vi "RT_W&R_ADC_W_DAC.vi"() -> ()   [LabVIEW 2018]
uses:
  <vilib>/Platform/TimedLoop/XDataNode/timing_clust.ctl
  <vilib>/Platform/TimedLoop/XDataNode/nitl_modes.ctl
  <vilib>/Platform/TimedLoop/XDataNode/wakeup.ctl
  <vilib>/FPGAPlugInAG/myRIO-1900/niLvFpga_Open_myRIO-1900.vi
  <vilib>/rvi/interface/common/dynamic/niFpgaDynamicAddResources.vi
  <vilib>/Utility/error.llb/Error Cluster From Error Code.vi
  <vilib>/rvi/errors/niLvFpgaAdjustHostInterfaceError.vi
  <vilib>/FPGAPlugInAG/Dynamic/niLvFpga_Close_Dynamic.vi
  <vilib>/Platform/TimedLoop/XDataNode/XDataNode.xnode
  <vilib>/rvi/interface/nirviOpenFPGA/nirviOpenFPGA.xnode
  ASPE_SC_Amp_HS/FPGA Bitfiles/ASPESCAmpControl_FPGATarget_FPGASPIW&RADCWDA_vR5pGZ7Mmx4.lvbitx
  FPGA_SPI_W&R_ADC_W_DACs.vi
  <vilib>/rvi/interface/nirviReadWriteControl/nirviReadWriteControl.xnode
  <vilib>/rvi/interface/nirviCloseFPGA/nirviCloseFPGA.xnode
  <vilib>/Platform/TimedLoop/XDataNode/XDNodeRunTimeDep.lvlib
  NiFpgaLv.dll
  <vilib>/rvi/interface/Simulation/niFpgaSimulationCallBeginRW.vi
panel:
  out "Loop rate (kHz)":dbl
  in  "Stop Button":bool
  in  "CH1":bool[](array[boolean])=[FALSE, FALSE, FALSE, FALSE, FALSE, TRUE, FALSE, FALSE, FALSE, FALSE, FALSE, FALSE, FALSE, FALSE, FALSE, FALSE]
  in  "CH4":bool[](array[boolean])=[FALSE, FALSE, TRUE, TRUE, FALSE, TRUE, FALSE, FALSE, FALSE, FALSE, FALSE, FALSE, FALSE, FALSE, FALSE, FALSE]
  in  "CH3":bool[](array[boolean])=[FALSE, FALSE, TRUE, FALSE, FALSE, TRUE, FALSE, FALSE, FALSE, FALSE, FALSE, FALSE, FALSE, FALSE, FALSE, FALSE]
  in  "CH2":bool[](array[boolean])=[FALSE, FALSE, FALSE, TRUE, FALSE, TRUE, FALSE, FALSE, FALSE, FALSE, FALSE, FALSE, FALSE, FALSE, FALSE, FALSE]
  out "ADC 4":dbl(graph)=-2.0281672948105642
  out "ADC 3":dbl(graph)=-0.5364908372369804
  out "ADC 2":dbl(graph)=-0.0015258556235409
  out "ADC 1":dbl(graph)=-0.0015258556235409
  in  "us":u32=150
  out "Finished Late? [i-1]":bool
  # "You can read the voltage ouput of sensors in the following plots"
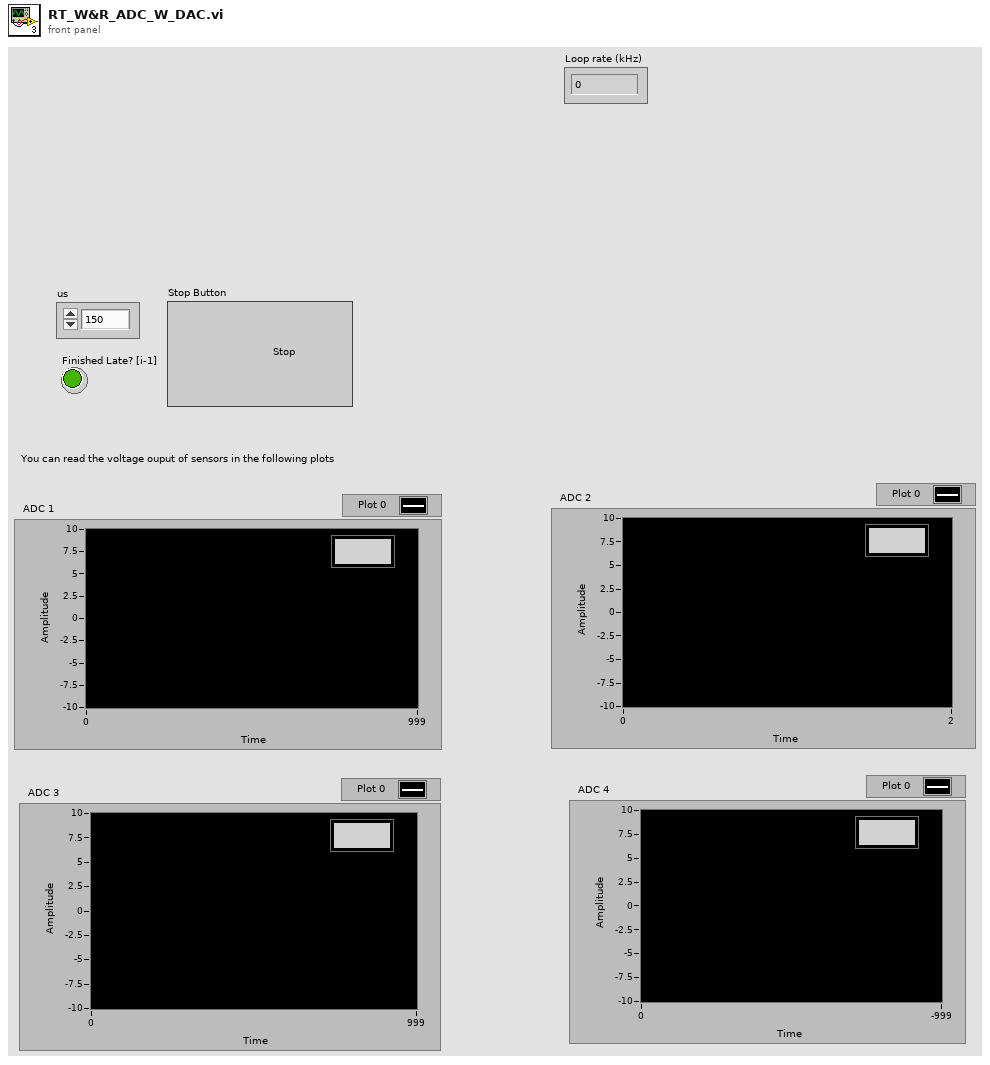
[diagram p1: front panel]
types:
  T1 = typedef "XDNodeRunTimeDep.lvlib/timing_clust.ctl" = cluster{"Expected End [f-1]":u64, "Actual End [f-1]":u64, "Finished Late? [f-1]":bool, "Expected End [i-1]":u64, "Actual End [i-1]":u64, "Finished Late? [i-1]":bool, "Expected Start [i]":u64, "Actual Start [i]":u64, "Expected Start [f]":u64, "Actual Start [f]":u64, "Source Name":string, "Structure Name":string, "Period":i64, "Deadline":i64, "Offset":i64, "Start":i64, "Priority":i32, "Timeout":i32, "Mode":T2, "Wakeup Reason":T3, "Error":errorcluster, "Source Type":string, "Secondary Source Type":string, "Global End Time":u64, "Global Start Time":u64, "Frame Duration":u64, "Iteration Duration":u64, "Assigned CPU":i32, "I/O Scan Engine Mode":u32}
  T2 = typedef "XDNodeRunTimeDep.lvlib/nitl_modes.ctl" = enum32{"No Change", "Process missed periods, maintain original phase", "Discard missed periods, maintain original phase", "Process missed periods, ignore original phase", "Discard missed periods, ignore original phase"}
  T3 = typedef "XDNodeRunTimeDep.lvlib/wakeup.ctl" = enum32{"Normal", "Aborted", "Asynchronous wakeup", "Timing source error", "Timed loop error", "Timeout"}
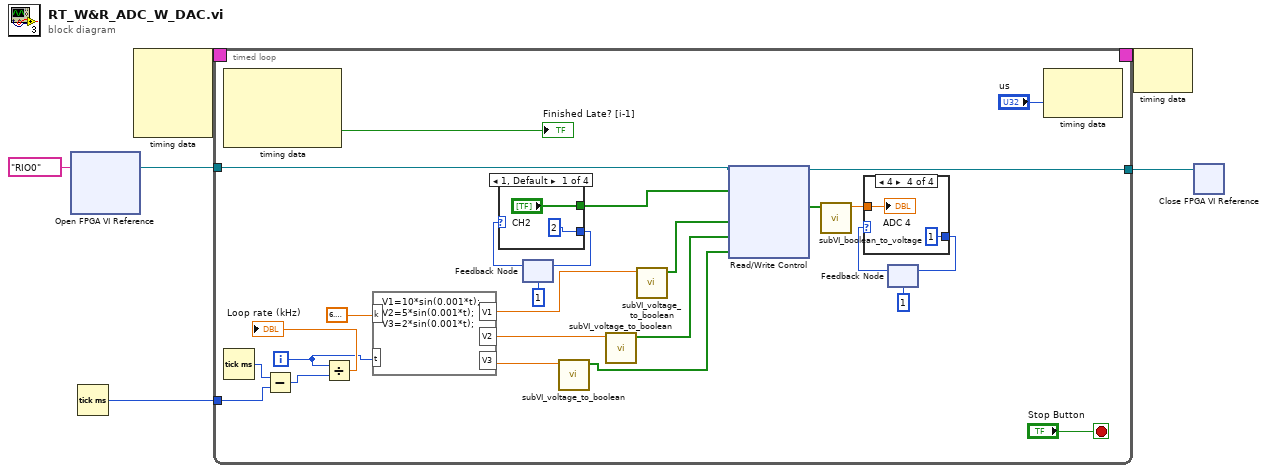
[diagram p0: block diagram]
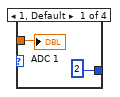
[diagram p2: hidden frame]
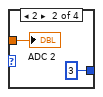
[diagram p3: hidden frame]
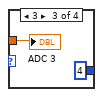
[diagram p4: hidden frame]
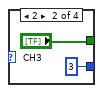
[diagram p5: hidden frame]
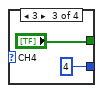
[diagram p6: hidden frame]
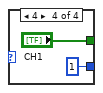
[diagram p7: hidden frame]
diagram:
  n1 = xnode "Open FPGA VI Reference"("resource name"=tag "RIO0") -> ("FPGA VI Reference Out"=w3:refnum<k20>)  [unwired: 1 in, 1 out]
  n2 = Tick Count (ms)() -> (millisecond timer value=w1:u32)
  n3 = node-c288() -> (w6:T1)  [unwired: 4 in]
  n4 = timed-loop {
    tunnel: w3 -> [w32]
    timing: w6 -> [_]
    timing-out: [_] -> w5
    tunnel: [w19] -> w4
    tunnel: w1 -> [w17]
    i -> [w13]
    stop <- "Stop Button" stop-if-true
    n5 = node-c288() -> (→"Finished Late? [i-1]":bool)  [unwired: 1 in, 3 out]
    n6 = Tick Count (ms)() -> (millisecond timer value=w18:u32)
    n7 = Subtract(x=w18, y=w17) -> (x-y=w14:u32)
    n8 = Divide(x=w13, y=w14) -> (x/y=→"Loop rate (kHz)":dbl)
    n9 = formula code="V1=10*sin(0.001*t);\nV2=5*sin(0.001*t);\nV3=2*sin(0.001*t);"("k"=6.283185307179586, "t"=w13) -> ("V1"=w11:dbl, "V2"=w10:dbl, "V3"=w8:dbl)
    n10 = feedback #1(1) -> (w30:i32)
    n11 = case shown="1, Default" w30 {
      tunnel: ["CH2" "CH3" "CH4" "CH1"] -> w27
      tunnel: [2 3 4 1] -> w28
      frame 1, Default {
      }
      frame 2 {
      }
      frame 3 {
      }
      frame 4 {
      }
    }
    n12 = feedback-in #1(w28) -> ()
    n13 = call "subVI_voltage_to_boolean.vi"("voltage"=w8) -> ("binary"=w7:bool[])  [unwired: 10 in]
    n14 = call "subVI_voltage_to_boolean.vi"("voltage"=w10) -> ("binary"=w9:bool[])  [unwired: 10 in]
    n15 = call "subVI_voltage_to_boolean.vi"("voltage"=w11) -> ("binary"=w12:bool[])  [unwired: 10 in]
    n16 = xnode "Read/Write Control"("FPGA VI Reference In"=w32, "ADC write"=w27, "DAC 1 write"=w12, "DAC 2 write"=w9, "DAC 3 write"=w7) -> ("FPGA VI Reference Out"=w19:refnum<k20>, "ADC read"=w20:bool[])  [unwired: 1 in, 1 out]
    n17 = call "subVI_boolean_to_voltage.vi"("ADC read"=w20) -> ("V"=w23:dbl)  [unwired: 10 in]
    n18 = feedback #2(1) -> (w26:i32)
    n19 = case shown="4" w26 {
      tunnel: [2 3 4 1] -> w24
      tunnel: w23 -> [w38 w40 w42 w44]
      frame 1, Default {
        "ADC 1" <- w38
      }
      frame 2 {
        "ADC 2" <- w40
      }
      frame 3 {
        "ADC 3" <- w42
      }
      frame 4 {
        "ADC 4" <- w44
      }
    }
    n20 = feedback-in #2(w24) -> ()
    n21 = node-c288("us") -> ()  [unwired: 1 in, 1 out]
  }
  n22 = node-c288(w5) -> ()  [unwired: 1 out]
  n23 = xnode "Close FPGA VI Reference"("FPGA VI Reference In"=w4) -> ()  [unwired: 1 in, 1 out]
